vi "check VI and controls in memory.vi"(8 "error in (no error) 2":errorcluster, 11 "Input command":string="Write to VISA, \u0000\u0000\u0000\u000eGPIB::12::inst, , offoff") -> (0 "error out":errorcluster, 1 "error message":string, 2 "Identifield command":string="Write to VISA", 3 "output command":string)   [LabVIEW 2025]
uses:
  <vilib>/Utility/error.llb/Trim Whitespace One-Sided.vi
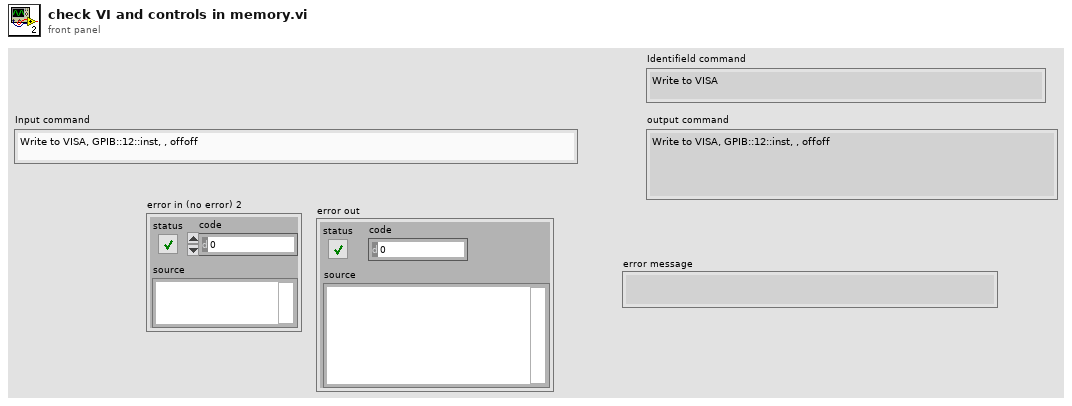
[diagram p1: front panel]
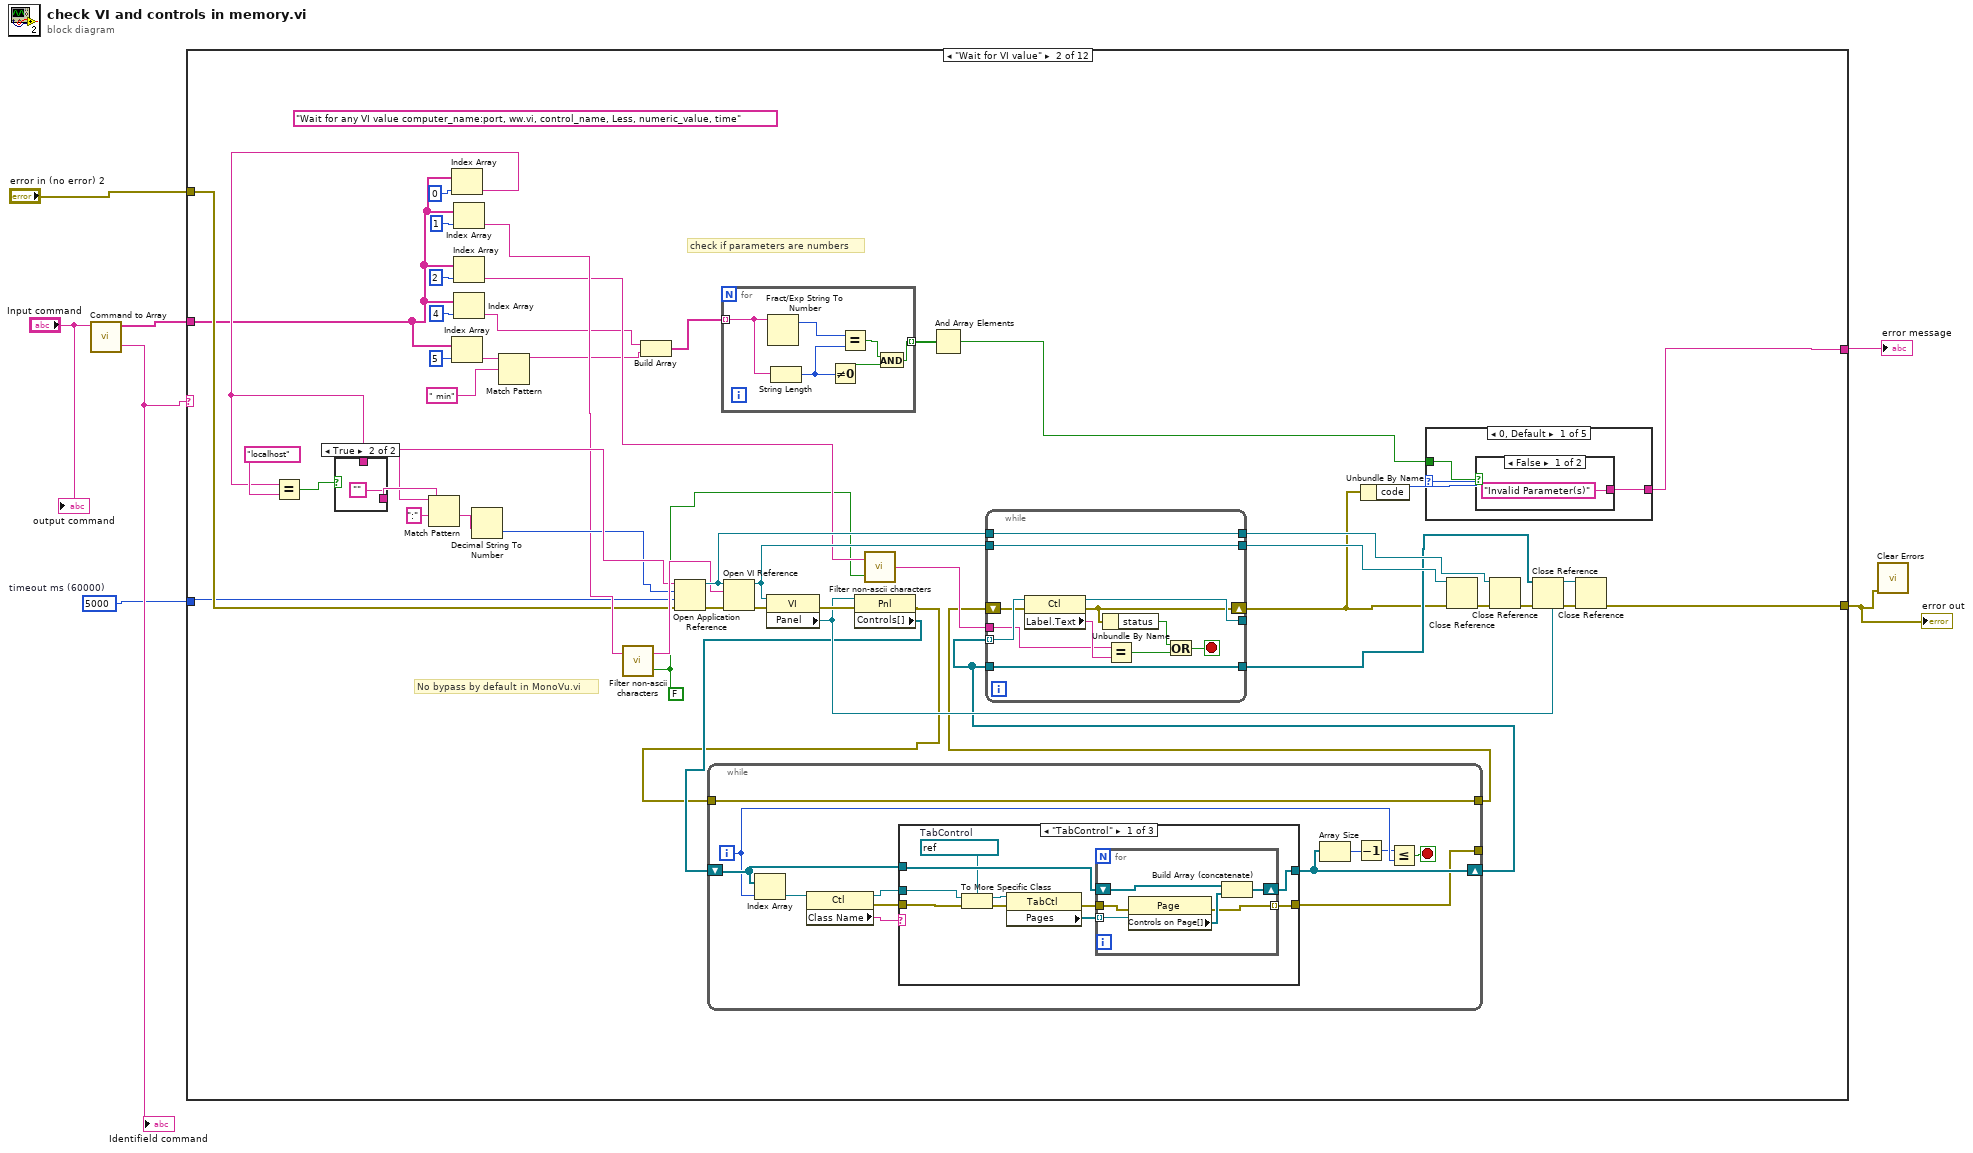
[diagram p0: block diagram]
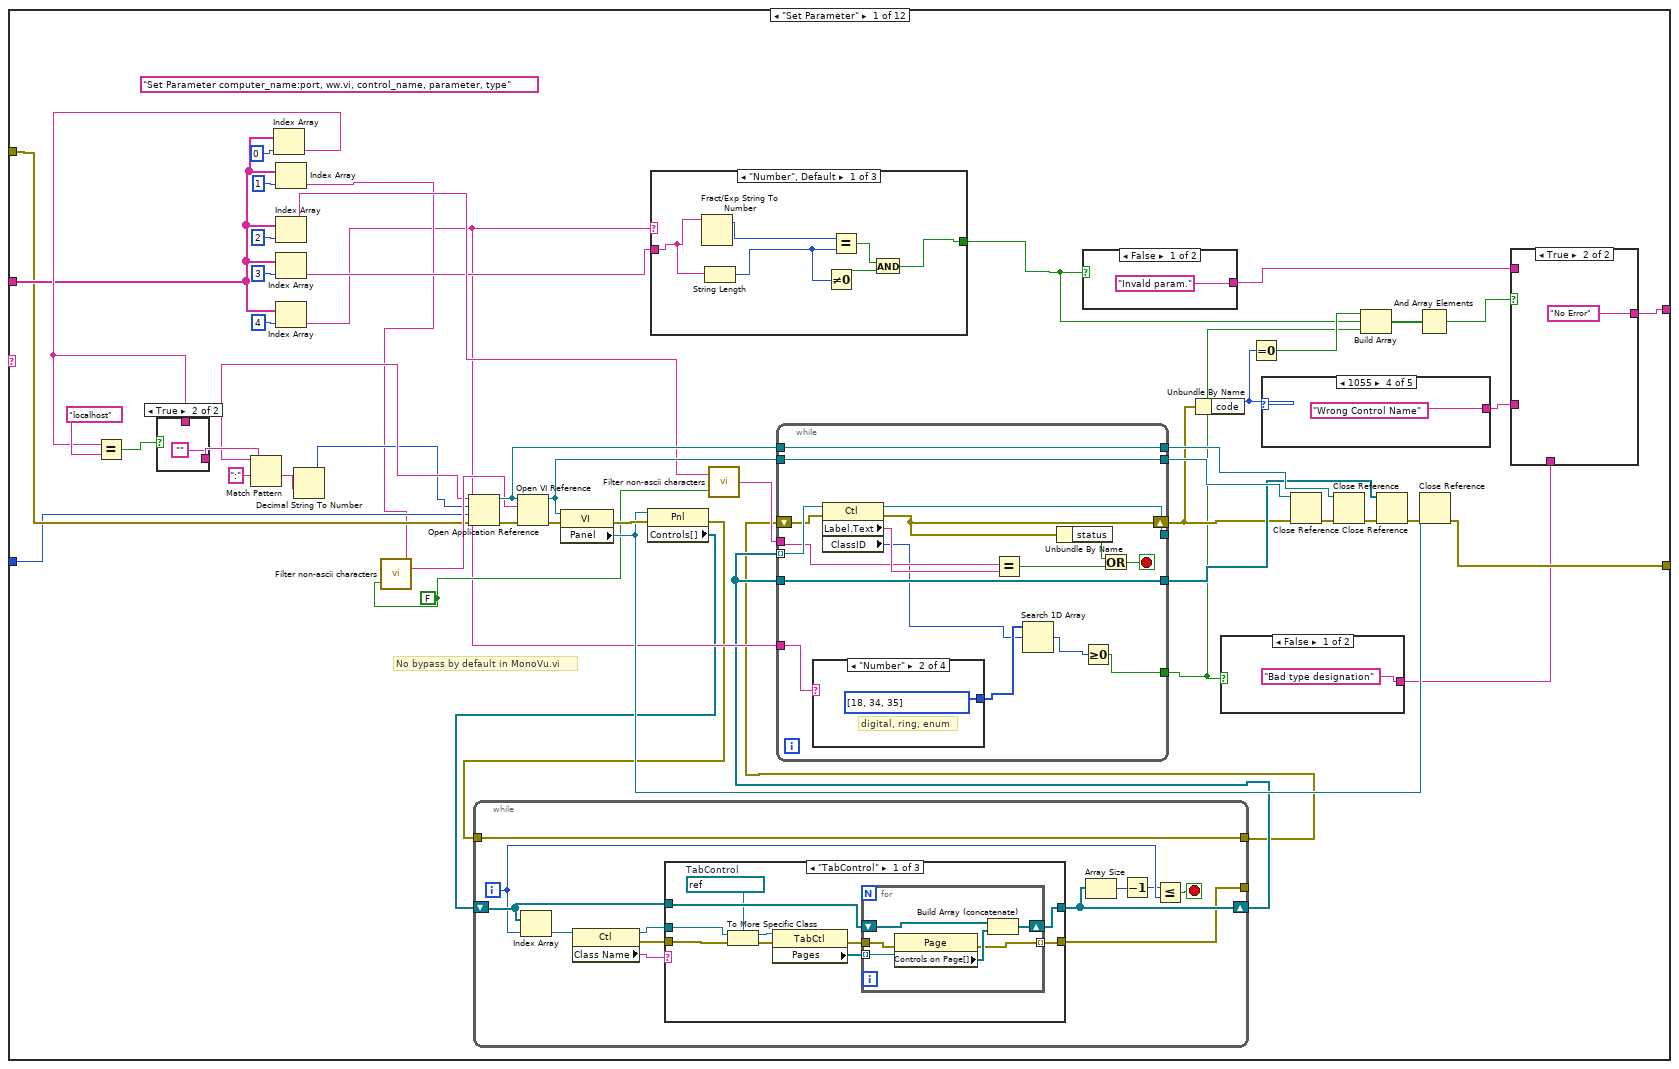
[diagram p2: hidden frame]
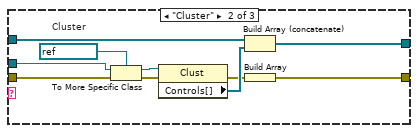
[diagram p3: hidden frame]
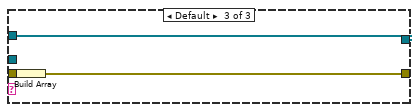
[diagram p4: hidden frame]
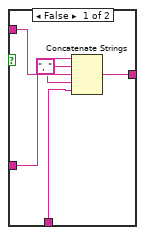
[diagram p5: hidden frame]
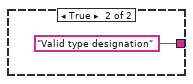
[diagram p6: hidden frame]
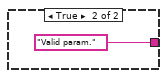
[diagram p7: hidden frame]
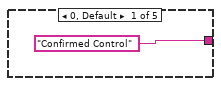
[diagram p8: hidden frame]
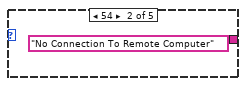
[diagram p9: hidden frame]
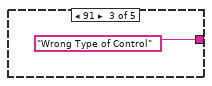
[diagram p10: hidden frame]
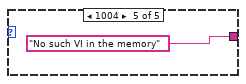
[diagram p11: hidden frame]
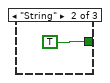
[diagram p12: hidden frame]
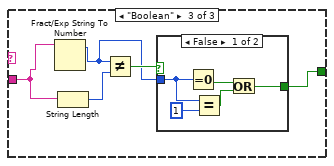
[diagram p13: hidden frame]
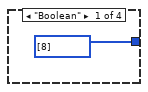
[diagram p16: hidden frame]
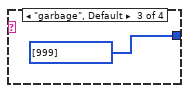
[diagram p17: hidden frame]
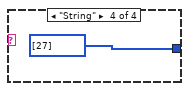
[diagram p18: hidden frame]
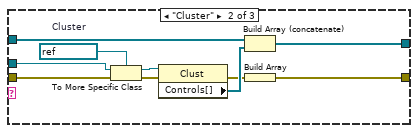
[diagram p19: hidden frame]
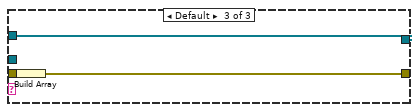
[diagram p20: hidden frame]
diagram:
  w1 = 5000  # timeout ms (60000)
  n1 = call "Command to Array.vi"("Input command"="Input command") -> ("parameter array"=w5:string[], "Identifield command"=w3:string)  [unwired: 8 in]
  "Identifield command" <- w3
  n2 = case shown="\"Wait for VI value\"" w3 {
    tunnel: [w43 w188 w280 w307 w330 w333 _ w435 w464 w499 w516 w527] -> w7
    tunnel: "error in (no error) 2" -> [w25 w170 w281 w308 w330 w335 w395 w436 w465 w499 w518 w527]
    tunnel: w5 -> [w26 w164 w283 w310 _ w345 w398 w439 w473 w493 w522 w537]
    tunnel: [w12 w171 w282 w309 "No Error" w346 w394 w437 w463 w495 w520 w528] -> w2
    tunnel: w1 -> [w24 w169 w279 w306 _ _ _ _ _ _ _ _]
    frame "Set Parameter" {
      (unwired) "Set Parameter computer_name:port, ww.vi, control_name, parameter, type" ("format string")
      w28 = FALSE ("bypass")
      # "No bypass by default in MonoVu.vi"
      n3 = Index Array(array=w26, index=0) -> (element=w32:string)
      n4 = Equal?(x=w32, y="localhost") -> (x = y?=w36:bool)
      n5 = case shown="True" w36 {
        tunnel: [w133 ""] -> w33
        tunnel: w32 -> [w133 _]
        frame False {
        }
        frame True {
        }
      }
      n6 = Match Pattern(string=w33, regular expression=":") -> (before substring=w31:string, after substring=w34:string)  [unwired: 1 in, 2 out]
      n7 = Index Array(array=w26, index=1) -> (element=w23:string)
      n8 = Index Array(array=w26, index=2) -> (element=w29:string)
      n9 = Index Array(array=w26, index=3) -> (element=w27:string)
      n10 = Index Array(array=w26, index=4) -> (element=w22:string)
      n11 = Decimal String To Number(string=w34) -> (number=w30:i32)  [unwired: 2 in, 1 out]
      n12 = call "Filter non-ascii characters.vi"("bypass"=w28, 2:w23) -> ("output"=w45:string)
      n13 = Open Application Reference(8:w25, 9:w24, 10:w30, 11:w31) -> (0:w56:errorcluster, 3:w53:refnum<vi>)
      n14 = Open VI Reference(application reference (local)=w53, vi path=w45, error in (no error)=w56) -> (vi reference=w55:refnum<vi>, error out=w58:errorcluster)  [unwired: 3 in]
      n15 = property class="VI"(reference=w55, error in=w58) -> (error out=w57:errorcluster, "Panel"=w46:refnum<vi>)  [unwired: 1 out]
      n16 = property class="Pnl"(reference=w46, error in=w57) -> (error out=w9:errorcluster, "Controls[]"=w11:refnum<vi>[])  [unwired: 1 out]
      n17 = while {
        shift-right: [w69] -> w10
        shift-left: w11 -> [w70]
        tunnel: [w60] -> _
        tunnel: w9 -> [w59]
        tunnel: [w59] -> w8
        i -> [w67]
        stop <- w66 stop-if-true
        n18 = Index Array(array=w70, index=w67) -> (element=w64:refnum<vi>)
        n19 = property class="Ctl"(reference=w64) -> (reference out=w62:refnum<vi>, error out=w61:errorcluster, "Class Name"=w63:string)  [unwired: 1 in]
        n20 = case shown="\"TabControl\"" w63 {
          tunnel: w70 -> [w79 w96 w99]
          tunnel: [w78 w95 w99] -> w69
          tunnel: w62 -> [w77 w94 _]
          tunnel: w61 -> [w76 w93 w98]
          tunnel: [w71 w87 w97] -> w60
          frame "TabControl" {
            w73 = refnum<vi> refnum  # TabControl
            n21 = To More Specific Class(target class=w73, reference=w77, error in=w76) -> (specific class reference=w74:refnum<vi>, error out=w75:errorcluster)
            n22 = property class="TabCtl"(reference=w74, error in=w75) -> (error out=w72:errorcluster, "Pages"=w80:refnum<vi>[])  [unwired: 1 out]
            n23 = for {
              tunnel: w80 -> [w86] mode=indexing
              shift-right: [w85] -> w78
              shift-left: w79 -> [w84]
              tunnel: w72 -> [w82]
              tunnel: [w81] -> w71 mode=indexing
              n24 = property class="Page"(reference=w86, error in=w82) -> (error out=w81:errorcluster, "Controls on Page[]"=w83:refnum<vi>[])  [unwired: 1 out]
              n25 = Build Array (concatenate)(w84, w83) -> (w85:refnum<vi>[])
            }
          }
          frame "Cluster" {
            w90 = refnum<vi> refnum  # Cluster
            n26 = To More Specific Class(target class=w90, reference=w94, error in=w93) -> (specific class reference=w91:refnum<vi>, error out=w92:errorcluster)
            n27 = property class="Clust"(reference=w91, error in=w92) -> (error out=w88:errorcluster, "Controls[]"=w89:refnum<vi>[])  [unwired: 1 out]
            n28 = Build Array (concatenate)(w96, w89) -> (w95:refnum<vi>[])
            n29 = Build Array(w88) -> (w87:errorcluster[])
          }
          frame Default {
            n30 = Build Array(w98) -> (w97:errorcluster[])
          }
        }
        n31 = Array Size(array=w69) -> (size(s)=w68:i32)
        n32 = Decrement(x=w68) -> (x-1=w65:i32)
        n33 = Less Or Equal?(x=w65, y=w67) -> (x <= y?=w66:bool)
      }
      n34 = case shown="\"Number\", Default" w22 {
        tunnel: w27 -> [w120 _ w125]
        tunnel: [w115 TRUE w122] -> w19
        frame "Number", Default {
          n35 = Fract/Exp String To Number(string=w120) -> (offset past number=w119:i32)  [unwired: 3 in, 1 out]
          n36 = String Length(string=w120) -> (length=w117:i32)
          n37 = Not Equal To 0?(x=w117) -> (x != 0?=w118:bool)
          n38 = Equal?(x=w119, y=w117) -> (x = y?=w116:bool)
          n39 = And(x=w116, y=w118) -> (x .and. y?=w115:bool)
        }
        frame "String" {
        }
        frame "Boolean" {
          n40 = Fract/Exp String To Number(string=w125) -> (offset past number=w123:i32)  [unwired: 3 in, 1 out]
          n41 = String Length(string=w125) -> (length=w126:i32)
          n42 = Not Equal?(x=w123, y=w126) -> (x != y?=w124:bool)
          n43 = case shown="False" w124 {
            selector: w124 -> [_ w132]
            tunnel: w123 -> [w131 _]
            tunnel: [w127 w132] -> w122
            frame False {
              n44 = Equal To 0?(x=w131) -> (x = 0?=w129:bool)
              n45 = Equal?(x=w131, y=1) -> (x = y?=w128:bool)
              n46 = Or(x=w129, y=w128) -> (x .or. y?=w127:bool)
            }
            frame True {
            }
          }
        }
      }
      n47 = call "Filter non-ascii characters.vi"("bypass"=w28, 2:w29) -> ("output"=w44:string)
      n48 = while {
        tunnel: w10 -> [w151] mode=indexing
        tunnel: w44 -> [w149]
        shift-right: [w146] -> w50
        shift-left: w8 -> [w148]
        tunnel: [w147] -> _
        tunnel: w55 -> [w142]
        tunnel: [w142] -> w54
        tunnel: w53 -> [w141]
        tunnel: [w141] -> w52
        tunnel: w10 -> [w140]
        tunnel: [w140] -> w51
        tunnel: w22 -> [w139]
        tunnel: [w135] -> w18
        stop <- w143 stop-if-true
        n49 = case shown="\"Number\"" w139 {
          tunnel: [u32[] [8] i32[] [18, 34, 35] u32[] [999] u32[] [27]] -> w138
          frame "Boolean" {
          }
          frame "Number" {
            # "digital, ring, enum"
          }
          frame "garbage", Default {
          }
          frame "String" {
          }
        }
        n50 = property class="Ctl"(reference=w151, error in=w148) -> (reference out=w147:refnum<vi>, error out=w146:errorcluster, "Label.Text"=w150:string, "ClassID"=w137:u32)
        n51 = Equal?(x=w149, y=w150) -> (x = y?=w144:bool)
        n52 = Search 1D Array(1D array=w138, element=w137) -> (index of element=w136:i32)  [unwired: 1 in]
        n53 = Unbundle By Name(w146) -> ("status"=w145:bool)
        n54 = Greater Or Equal To 0?(x=w136) -> (x >= 0?=w135:bool)
        n55 = Or(x=w145, y=w144) -> (x .or. y?=w143:bool)
      }
      n56 = case shown="False" w19 {
        tunnel: ["Invald param." ("Control Name") "Valid param." ("Control Name")] -> w14
        frame False {
        }
        frame True {
        }
      }
      n57 = Unbundle By Name(w50) -> ("code"=w21:i32)
      n58 = case shown="False" w18 {
        tunnel: ["Bad type designation" ("Control Name") "Valid type designation" ("Control Name")] -> w13
        frame False {
        }
        frame True {
        }
      }
      n59 = Equal To 0?(x=w21) -> (x = 0?=w20:bool)
      n60 = case shown="1055" w21 {
        tunnel: ["Confirmed Control" ("Control Name") "No Connection To Remote Computer" ("Control Name") "Wrong Type of Control" ("Control Name") "Wrong Control Name" ("Control Name") "No such VI in the memory" ("Control Name")] -> w15
        frame 0, Default {
        }
        frame 54 {
        }
        frame 91 {
        }
        frame 1055 {
        }
        frame 1004 {
        }
      }
      n61 = Close Reference(reference=w54, error in (no error)=w50) -> (error out=w49:errorcluster)
      n62 = Close Reference(reference=w52, error in (no error)=w49) -> (error out=w48:errorcluster)
      n63 = Build Array(w20, w19, w18) -> (w17:bool[])
      n64 = Close Reference(reference=w51, error in (no error)=w48) -> (error out=w47:errorcluster)
      n65 = And Array Elements(Boolean array=w17) -> (logical AND=w16:bool)
      n66 = Close Reference(reference=w46, error in (no error)=w47) -> (error out=w43:errorcluster)
      n67 = case shown="True" w16 {
        tunnel: w15 -> [w104 _]
        tunnel: w14 -> [w103 _]
        tunnel: w13 -> [w101 _]
        tunnel: [w100 "No Error"] -> w12
        frame False {
          w102 = ", " ("string")
          n68 = Concatenate Strings(w104, w102, w103, w102, w101) -> (w100:string)
        }
        frame True {
        }
      }
    }
    frame "Wait for VI value" {
      (unwired) "Wait for any VI value computer_name:port, ww.vi, control_name, Less, numeric_value, time" ("format string")
      w172 = FALSE ("bypass")
      # "check if parameters are numbers"
      # "No bypass by default in MonoVu.vi"
      n69 = Index Array(array=w164, index=0) -> (element=w178:string)
      n70 = Equal?(x=w178, y="localhost") -> (x = y?=w182:bool)
      n71 = case shown="True" w182 {
        tunnel: [w259 ""] -> w179
        tunnel: w178 -> [w259 _]
        frame False {
        }
        frame True {
        }
      }
      n72 = Match Pattern(string=w179, regular expression=":") -> (before substring=w177:string, after substring=w180:string)  [unwired: 1 in, 2 out]
      n73 = Index Array(array=w164, index=5) -> (element=w162:string)
      n74 = Index Array(array=w164, index=1) -> (element=w175:string)
      n75 = Index Array(array=w164, index=2) -> (element=w174:string)
      n76 = Index Array(array=w164, index=4) -> (element=w168:string)
      n77 = Decimal String To Number(string=w180) -> (number=w176:i32)  [unwired: 2 in, 1 out]
      n78 = Match Pattern(string=w162, regular expression=" min") -> (before substring=w160:string)  [unwired: 1 in, 3 out]
      n79 = call "Filter non-ascii characters.vi"("bypass"=w172, 2:w175) -> ("output"=w190:string)
      n80 = Build Array(w168, w160) -> (w167:string[])
      n81 = Open Application Reference(8:w170, 9:w169, 10:w176, 11:w177) -> (0:w201:errorcluster, 3:w198:refnum<vi>)
      n82 = for {
        tunnel: [w246] -> w166 mode=indexing
        tunnel: w167 -> [w245] mode=indexing
        n83 = Fract/Exp String To Number(string=w245) -> (offset past number=w250:i32)  [unwired: 3 in, 1 out]
        n84 = String Length(string=w245) -> (length=w249:i32)
        n85 = Not Equal To 0?(x=w249) -> (x != 0?=w248:bool)
        n86 = Equal?(x=w250, y=w249) -> (x = y?=w247:bool)
        n87 = And(x=w247, y=w248) -> (x .and. y?=w246:bool)
      }
      n88 = Open VI Reference(application reference (local)=w198, vi path=w190, error in (no error)=w201) -> (vi reference=w200:refnum<vi>, error out=w203:errorcluster)  [unwired: 3 in]
      n89 = property class="VI"(reference=w200, error in=w203) -> (error out=w202:errorcluster, "Panel"=w191:refnum<vi>)  [unwired: 1 out]
      n90 = property class="Pnl"(reference=w191, error in=w202) -> (error out=w158:errorcluster, "Controls[]"=w159:refnum<vi>[])  [unwired: 1 out]
      n91 = while {
        shift-right: [w214] -> w156
        shift-left: w159 -> [w215]
        tunnel: [w205] -> _
        tunnel: w158 -> [w204]
        tunnel: [w204] -> w157
        i -> [w212]
        stop <- w211 stop-if-true
        n92 = Index Array(array=w215, index=w212) -> (element=w209:refnum<vi>)
        n93 = property class="Ctl"(reference=w209) -> (reference out=w207:refnum<vi>, error out=w206:errorcluster, "Class Name"=w208:string)  [unwired: 1 in]
        n94 = case shown="\"TabControl\"" w208 {
          tunnel: w215 -> [w224 w241 w244]
          tunnel: [w223 w240 w244] -> w214
          tunnel: w207 -> [w222 w239 _]
          tunnel: w206 -> [w221 w238 w243]
          tunnel: [w216 w232 w242] -> w205
          frame "TabControl" {
            w218 = refnum<vi> refnum  # TabControl
            n95 = To More Specific Class(target class=w218, reference=w222, error in=w221) -> (specific class reference=w219:refnum<vi>, error out=w220:errorcluster)
            n96 = property class="TabCtl"(reference=w219, error in=w220) -> (error out=w217:errorcluster, "Pages"=w225:refnum<vi>[])  [unwired: 1 out]
            n97 = for {
              tunnel: w225 -> [w231] mode=indexing
              shift-right: [w230] -> w223
              shift-left: w224 -> [w229]
              tunnel: w217 -> [w227]
              tunnel: [w226] -> w216 mode=indexing
              n98 = property class="Page"(reference=w231, error in=w227) -> (error out=w226:errorcluster, "Controls on Page[]"=w228:refnum<vi>[])  [unwired: 1 out]
              n99 = Build Array (concatenate)(w229, w228) -> (w230:refnum<vi>[])
            }
          }
          frame "Cluster" {
            w235 = refnum<vi> refnum  # Cluster
            n100 = To More Specific Class(target class=w235, reference=w239, error in=w238) -> (specific class reference=w236:refnum<vi>, error out=w237:errorcluster)
            n101 = property class="Clust"(reference=w236, error in=w237) -> (error out=w233:errorcluster, "Controls[]"=w234:refnum<vi>[])  [unwired: 1 out]
            n102 = Build Array (concatenate)(w241, w234) -> (w240:refnum<vi>[])
            n103 = Build Array(w233) -> (w232:errorcluster[])
          }
          frame Default {
            n104 = Build Array(w243) -> (w242:errorcluster[])
          }
        }
        n105 = Array Size(array=w214) -> (size(s)=w213:i32)
        n106 = Decrement(x=w213) -> (x-1=w210:i32)
        n107 = Less Or Equal?(x=w210, y=w212) -> (x <= y?=w211:bool)
      }
      n108 = call "Filter non-ascii characters.vi"("bypass"=w172, 2:w174) -> ("output"=w189:string)
      n109 = And Array Elements(Boolean array=w166) -> (logical AND=w165:bool)
      n110 = while {
        tunnel: w156 -> [w272] mode=indexing
        tunnel: w189 -> [w270]
        shift-right: [w267] -> w195
        shift-left: w157 -> [w269]
        tunnel: [w268] -> _
        tunnel: w200 -> [w263]
        tunnel: [w263] -> w199
        tunnel: w198 -> [w262]
        tunnel: [w262] -> w197
        tunnel: w156 -> [w261]
        tunnel: [w261] -> w196
        stop <- w264 stop-if-true
        n111 = property class="Ctl"(reference=w272, error in=w269) -> (reference out=w268:refnum<vi>, error out=w267:errorcluster, "Label.Text"=w271:string)
        n112 = Unbundle By Name(w267) -> ("status"=w266:bool)
        n113 = Equal?(x=w270, y=w271) -> (x = y?=w265:bool)
        n114 = Or(x=w266, y=w265) -> (x .or. y?=w264:bool)
      }
      n115 = Unbundle By Name(w195) -> ("code"=w173:i32)
      n116 = case shown="0, Default" w173 {
        tunnel: [w252 "No Connection To Remote Computer" ("Control Name") "Wrong Type of Control" ("Control Name") "Wrong Control Name" ("Control Name") "No such VI in the memory" ("Control Name")] -> w171
        tunnel: w165 -> [w251 _ _ _ _]
        frame 0, Default {
          n117 = case shown="False" w251 {
            tunnel: ["Invalid Parameter(s)" ("Control Name") "No Error" ("Control Name")] -> w252
            frame False {
            }
            frame True {
            }
          }
        }
        frame 54 {
        }
        frame 91 {
        }
        frame 1055 {
        }
        frame 1004 {
        }
      }
      n118 = Close Reference(reference=w199, error in (no error)=w195) -> (error out=w194:errorcluster)
      n119 = Close Reference(reference=w197, error in (no error)=w194) -> (error out=w193:errorcluster)
      n120 = Close Reference(reference=w196, error in (no error)=w193) -> (error out=w192:errorcluster)
      n121 = Close Reference(reference=w191, error in (no error)=w192) -> (error out=w188:errorcluster)
    }
    frame "Run VI" {
      (unwired) "Run VI: computer_name:port, ww.vi" ("format string")
      # "No bypass by default in MonoVu.vi"
      n122 = Index Array(array=w283, index=0) -> (element=w288:string)
      n123 = Equal?(x=w288, y="localhost") -> (x = y?=w292:bool)
      n124 = case shown="True" w292 {
        tunnel: [w299 ""] -> w289
        tunnel: w288 -> [w299 _]
        frame False {
        }
        frame True {
        }
      }
      n125 = Match Pattern(string=w289, regular expression=":") -> (before substring=w287:string, after substring=w290:string)  [unwired: 1 in, 2 out]
      n126 = Index Array(array=w283, index=1) -> (element=w275:string)
      n127 = Decimal String To Number(string=w290) -> (number=w286:i32)  [unwired: 2 in, 1 out]
      n128 = call "Filter non-ascii characters.vi"("bypass"=FALSE, 2:w275) -> ("output"=w273:string)
      n129 = Open Application Reference(8:w281, 9:w279, 10:w286, 11:w287) -> (0:w277:errorcluster, 3:w278:refnum<vi>)
      n130 = Open VI Reference(application reference (local)=w278, vi path=w273, error in (no error)=w277) -> (vi reference=w276:refnum<vi>, error out=w274:errorcluster)  [unwired: 3 in]
      n131 = Unbundle By Name(w274) -> ("code"=w285:i32)
      n132 = case shown="0, Default" w285 {
        tunnel: ["No Error" ("Control Name") "No Connection To Remote Computer" ("Control Name") "No such VI in the memory" ("Control Name")] -> w282
        frame 0, Default {
        }
        frame 54 {
        }
        frame 1004 {
        }
      }
      n133 = Close Reference(reference=w276, error in (no error)=w274) -> (error out=w280:errorcluster)
    }
    frame "Abort VI" {
      (unwired) "Abort VI: computer_name:port, ww.vi" ("format string")
      # "No bypass by default in MonoVu.vi"
      n134 = Index Array(array=w310, index=0) -> (element=w316:string)
      n135 = Equal?(x=w316, y="localhost") -> (x = y?=w320:bool)
      n136 = case shown="True" w320 {
        tunnel: [w327 ""] -> w317
        tunnel: w316 -> [w327 _]
        frame False {
        }
        frame True {
        }
      }
      n137 = Match Pattern(string=w317, regular expression=":") -> (before substring=w315:string, after substring=w318:string)  [unwired: 1 in, 2 out]
      n138 = Index Array(array=w310, index=1) -> (element=w313:string)
      n139 = Decimal String To Number(string=w318) -> (number=w314:i32)  [unwired: 2 in, 1 out]
      n140 = call "Filter non-ascii characters.vi"("bypass"=FALSE, 2:w313) -> ("output"=w301:string)
      n141 = Open Application Reference(8:w308, 9:w306, 10:w314, 11:w315) -> (0:w305:errorcluster, 3:w303:refnum<vi>)
      n142 = Open VI Reference(application reference (local)=w303, vi path=w301, error in (no error)=w305) -> (vi reference=w302:refnum<vi>, error out=w304:errorcluster)  [unwired: 3 in]
      n143 = Unbundle By Name(w304) -> ("code"=w312:i32)
      n144 = Close Reference(reference=w302, error in (no error)=w304) -> (error out=w307:errorcluster)
      n145 = case shown="1004" w312 {
        tunnel: ["No Error" ("Control Name") "No Connection To Remote Computer" ("Control Name") "No such VI in the memory" ("Control Name")] -> w309
        frame 0, Default {
        }
        frame 54 {
        }
        frame 1004 {
        }
      }
    }
    frame "anything else", Default {
    }
    frame "Set Temperature" {
      # "Set Temperature %s ( %s ) %s K at %s K/min, Output %s"
      # "Set Temperature LS336 ( GPIB::12::INSTR ) 23 K at 1 K/min, Output 1"
      n146 = Index Array(array=w345, index #1=1 ("index"), index #2=0 ("index")) -> (element #1=w334:string, element #2=w336:string)
      n147 = Array Subset(array=w345, index=2, length=2) -> (w344:string[])
      n148 = call <vilib>:"Trim Whitespace.vi"("string"=w336) -> ("trimmed string"=w339:string)  [unwired: 1 in]
      n149 = Not Equal?(x=w339, y="PPMS") -> (x != y?=w331:bool)
      n150 = case shown="False" w331 {
        tunnel: w335 -> [_ w361]
        tunnel: w334 -> [_ w360]
        tunnel: [w349 w356] -> w332
        tunnel: [w348 w355] -> w333
        frame False {
          n151 = Open VI Reference(vi path="PS Control.vi" ("y")) -> (vi reference=w350:refnum<vi>, error out=w351:errorcluster)  [unwired: 5 in]
          n152 = Close Reference(reference=w350, error in (no error)=w351) -> (error out=w348:errorcluster)
          n153 = case shown="No Error" w348 {
            tunnel: [0 2] -> w349
            frame No Error {
            }
            frame Error {
            }
          }
        }
        frame True {
          n154 = call "Check VISA instrument.vi"("error in (no error)"=w361, "visa instrumnet string"=w360) -> ("error out"=w355:errorcluster, "error"=w359:bool)  [unwired: 8 in]
          n155 = Equal?(x=w359, y=FALSE) -> (x = y?=w357:bool)
          n156 = case shown="False" w357 {
            tunnel: [1 0] -> w356
            frame False {
            }
            frame True {
            }
          }
        }
      }
      n157 = for {
        tunnel: w344 -> [w380] mode=indexing
        tunnel: [w376] -> w341 mode=indexing
        n158 = Fract/Exp String To Number(string=w380) -> (offset past number=w381:i32)  [unwired: 3 in, 1 out]
        n159 = String Length(string=w380) -> (length=w379:i32)
        n160 = Not Equal To 0?(x=w379) -> (x != 0?=w378:bool)
        n161 = Equal?(x=w381, y=w379) -> (x = y?=w377:bool)
        n162 = And(x=w377, y=w378) -> (x .and. y?=w376:bool)
      }
      n163 = And Array Elements(Boolean array=w341) -> (logical AND=w340:bool)
      n164 = case shown="True" w340 {
        tunnel: [w366 w371] -> w346
        tunnel: w332 -> [w365 w372]
        frame False {
          n165 = case shown="2" w365 {
            tunnel: ["" ", Invalid GPIB address" ", PS Control.vi is missing"] -> w364
            frame 0, Default {
            }
            frame 1 {
            }
            frame 2 {
            }
          }
          n166 = Concatenate Strings("Invalid Parameter(s)" ("string"), w364) -> (w366:string)
        }
        frame True {
          n167 = case shown="0, Default" w372 {
            tunnel: ["No Error" ", Invalid GPIB address" ", PS Control.vi is missing"] -> w371
            frame 0, Default {
            }
            frame 1 {
            }
            frame 2 {
            }
          }
        }
      }
    }
    frame "Wait for Temperature" {
      (unwired) "Wait for Temperature %s than %s K Sensor %s of %s ( %s ) Timeout %s min" ("format string")
      n168 = Index Array(array=w398, index #1=1 ("index"), index #2=5 ("index"), index #3=4 ("index"), index #4=3 ("index")) -> (element #1=w393:string, element #2=w390:string, element #3=w387:string, element #4=w382:string)
      n169 = call <vilib>:"Trim Whitespace.vi"("string"=w382) -> ("trimmed string"=w388:string)  [unwired: 1 in]
      n170 = Build Array(w393, w390) -> (w389:string[])
      n171 = Not Equal?(x=w388, y="PPMS") -> (x != y?=w385:bool)
      n172 = for {
        tunnel: [w428] -> w397 mode=indexing
        tunnel: w389 -> [w427] mode=indexing
        n173 = Fract/Exp String To Number(string=w427) -> (offset past number=w432:i32)  [unwired: 3 in, 1 out]
        n174 = String Length(string=w427) -> (length=w431:i32)
        n175 = Not Equal To 0?(x=w431) -> (x != 0?=w430:bool)
        n176 = Equal?(x=w432, y=w431) -> (x = y?=w429:bool)
        n177 = And(x=w429, y=w430) -> (x .and. y?=w428:bool)
      }
      n178 = case shown="True" w385 {
        tunnel: w395 -> [_ w412]
        tunnel: w387 -> [_ w411]
        tunnel: [w400 w407] -> w384
        frame False {
          n179 = Open VI Reference(vi path="PS Control.vi" ("y")) -> (vi reference=w402:refnum<vi>, error out=w403:errorcluster)  [unwired: 5 in]
          n180 = Close Reference(reference=w402, error in (no error)=w403) -> (error out=w401:errorcluster)
          n181 = case shown="Error .." w401 {
            tunnel: [0 2] -> w400
            frame No Error {
            }
            frame Error {
            }
          }
        }
        frame True {
          n182 = call "Check VISA instrument.vi"("error in (no error)"=w412, "visa instrumnet string"=w411) -> ("error"=w410:bool)  [unwired: 8 in, 1 out]
          n183 = Equal?(x=w410, y=FALSE) -> (x = y?=w408:bool)
          n184 = case shown="False" w408 {
            tunnel: [1 0] -> w407
            frame False {
            }
            frame True {
            }
          }
        }
      }
      n185 = And Array Elements(Boolean array=w397) -> (logical AND=w396:bool)
      n186 = case shown="True" w396 {
        tunnel: [w415 w422] -> w394
        tunnel: w384 -> [w416 w423]
        frame False {
          n187 = case shown="0, Default" w416 {
            tunnel: ["" ", Invalid GPIB address" ", PS Control.vi is missing"] -> w418
            frame 0, Default {
            }
            frame 1 {
            }
            frame 2 {
            }
          }
          n188 = Concatenate Strings("Invalid Parameter(s)" ("string"), w418) -> (w415:string)
        }
        frame True {
          n189 = case shown="1" w423 {
            tunnel: ["No Error" ", Invalid GPIB address" ", PS Control.vi is missing"] -> w422
            frame 0, Default {
            }
            frame 1 {
            }
            frame 2 {
            }
          }
        }
      }
    }
    frame "Set" {
      (unwired) "Set %s ( %s ) %s %s" ("format string")
      n190 = Index Array(array=w439, index=0) -> (element=w433:string)
      n191 = Index Array(array=w439, index=1) -> (element=w434:string)
      n192 = Index Array(array=w439, index=2) -> ()  [unwired: 1 out]
      n193 = Index Array(array=w439, index=3) -> ()  [unwired: 1 out]
      n194 = case shown="\"MotorControl\"" w433 {
        tunnel: [w447 w460] -> w437
        tunnel: w434 -> [w443 w459]
        tunnel: w436 -> [w445 w457]
        tunnel: [w444 w456] -> w435
        frame "MotorControl" {
          n195 = case shown="\"BLM\", Default" w443 {
            tunnel: ["Stepper Mover.vi" ("Target VI name") "BLM_ManualControl.vi" ("Target VI name")] -> w446
            frame "IMS" {
            }
            frame "BLM", Default {
            }
          }
          n196 = Open VI Reference(vi path=w446, error in (no error)=w445) -> (vi reference=w449:refnum<vi>, error out=w448:errorcluster)  [unwired: 4 in]
          n197 = Unbundle By Name(w448) -> ("code"=w450:i32)
          n198 = Close Reference(reference=w449, error in (no error)=w448) -> (error out=w444:errorcluster)
          n199 = case shown="0, Default" w450 {
            tunnel: ["No Error" ("Control Name") "No Connection To Remote Computer" ("Control Name") "No such VI in the memory" ("Control Name")] -> w447
            frame 0, Default {
            }
            frame 54 {
            }
            frame 1004 {
            }
          }
        }
        frame "Default", Default {
          n200 = call "Check VISA instrument.vi"("error in (no error)"=w457, "visa instrumnet string"=w459) -> ("error out"=w456:errorcluster, "error"=w458:bool)  [unwired: 8 in]
          n201 = case shown="True" w458 {
            tunnel: ["No Error" "Invalid GPIB address"] -> w460
            frame False {
            }
            frame True {
            }
          }
        }
      }
    }
    frame "Sweep" {
      (unwired) "Sweep %s ( %s ) Initial: %s mA Final: %s mA Period: %s min %s" ("format string")
      n202 = Index Array(array=w473, index=1) -> (element=w466:string)
      n203 = Array Subset(array=w473, index=2, length=3) -> (w467:string[])
      n204 = for {
        tunnel: w467 -> [w489] mode=indexing
        tunnel: [w485] -> w469 mode=indexing
        n205 = Fract/Exp String To Number(string=w489) -> (offset past number=w490:i32)  [unwired: 3 in, 1 out]
        n206 = String Length(string=w489) -> (length=w488:i32)
        n207 = Not Equal To 0?(x=w488) -> (x != 0?=w487:bool)
        n208 = Equal?(x=w490, y=w488) -> (x = y?=w486:bool)
        n209 = And(x=w486, y=w487) -> (x .and. y?=w485:bool)
      }
      n210 = call "Check VISA instrument.vi"("error in (no error)"=w465, "visa instrumnet string"=w466) -> ("error out"=w464:errorcluster, "error"=w470:bool)  [unwired: 8 in]
      n211 = And Array Elements(Boolean array=w469) -> (logical AND=w468:bool)
      n212 = case shown="True" w468 {
        tunnel: [w475 w482] -> w463
        tunnel: w470 -> [w476 w481]
        frame False {
          n213 = case shown="True" w476 {
            tunnel: ["" ", Invalid GPIB address"] -> w478
            frame False {
            }
            frame True {
            }
          }
          n214 = Concatenate Strings("Invalid Parameter(s)" ("string"), w478) -> (w475:string)
        }
        frame True {
          n215 = case shown="True" w481 {
            tunnel: ["No Error" "Invalid GPIB address"] -> w482
            frame False {
            }
            frame True {
            }
          }
        }
      }
    }
    frame "Set Field" {
      (unwired) "Set Field %s T at %s T/min" ("format string")
      n216 = for {
        tunnel: w493 -> [w504] mode=indexing
        tunnel: [w500] -> w492 mode=indexing
        n217 = Fract/Exp String To Number(string=w504) -> (offset past number=w505:i32)  [unwired: 3 in, 1 out]
        n218 = String Length(string=w504) -> (length=w503:i32)
        n219 = Not Equal To 0?(x=w503) -> (x != 0?=w502:bool)
        n220 = Equal?(x=w505, y=w503) -> (x = y?=w501:bool)
        n221 = And(x=w501, y=w502) -> (x .and. y?=w500:bool)
      }
      n222 = Index Array(array=w493, index=1) -> (element=w494:string)
      n223 = Fract/Exp String To Number(string=w494) -> (number=w497:dbl)  [unwired: 3 in, 1 out]
      n224 = Equal To 0?(x=w497) -> (x = 0?=w496:bool)
      n225 = And Array Elements(Boolean array=w492) -> (logical AND=w491:bool)
      n226 = case shown="False" w491 {
        tunnel: w496 -> [w509 w513]
        tunnel: [w506 w512] -> w495
        frame False {
          n227 = case shown="False" w509 {
            tunnel: ["" ", Invalid ramp rate"] -> w507
            frame False {
            }
            frame True {
            }
          }
          n228 = Concatenate Strings("Invalid Parameter(s)", w507) -> (w506:string)
        }
        frame True {
          n229 = case shown="False" w513 {
            tunnel: ["No Error" "Invalid ramp rate"] -> w512
            frame False {
            }
            frame True {
            }
          }
        }
      }
    }
    frame "Write to VISA" {
      n230 = Index Array(array=w522, index=0) -> (element=w519:string)
      n231 = Index Array(array=w522, index=1) -> ()  [unwired: 1 out]
      n232 = call "Check VISA instrument.vi"("error in (no error)"=w518, "visa instrumnet string"=w519) -> ("error out"=w516:errorcluster, "error"=w517:bool)  [unwired: 8 in]
      n233 = case shown="True" w517 {
        tunnel: ["No Error" "Invalid VISA reference"] -> w520
        frame False {
        }
        frame True {
        }
      }
    }
    frame "Wait for" {
      # "Warning message is not implemented"
      n234 = Index Array(array=w537, index=0) -> (element=w533:string)
      n235 = Index Array(array=w537, index=1) -> (element=w536:string)
      n236 = To Lower Case(string=w536) -> (all lower case string=w534:string)
      n237 = Fract/Exp String To Number(string=w533) -> (number=w532:dbl)  [unwired: 3 in, 1 out]
      n238 = Equal?(x=w534, y="hour") -> (x = y?=w529:bool)
      n239 = Greater Or Equal?(x=w532, y=2.0) -> (x >= y?=w530:bool)
      n240 = And(x=w530, y=w529) -> ()  [unwired: 1 out]
      n241 = case shown="True" FALSE {
        tunnel: ["No Error" ("Control Name") "Warning: long waiting " ("Control Name")] -> w528
        frame False {
        }
        frame True {
        }
      }
    }
  }
  "error out" <- w7
  "error message" <- w2
  n242 = call <vilib>:"Clear Errors.vi"("error in (no error)"=w7) -> ()  [unwired: 5 in, 2 out]
  "output command" <- "Input command"
